vi "ARN Auswertung.vi"(8 "error in (no error)":errorcluster caption="Fehler (Eingang, kein Fehler)") -> (0 "error out":errorcluster caption="Fehler (Ausgang)")   [LabVIEW 2020, in "EPA 1065.lvlib" / "ARN Test 1065-305.lvlib"]
uses:
  ARN Test 1065-305.lvlib
  Aktion FGV ARN Daten.ctl
  Messdaten/Gewichtung (Stichprobe).ctl
  Messdaten/Messdaten.lvlib
  ARN Modus.ctl
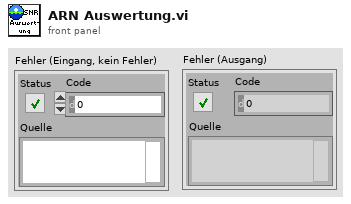
[diagram p1: front panel]
types:
  T1 = typedef "Messdaten.lvlib/Gewichtung (Stichprobe).ctl" = enum16{"Sample", "Population"}
  T2 = typedef "EPA 1065.lvlib/ARN Test 1065-305.lvlib/Aktion FGV ARN Daten.ctl" = enum16{"Lesen", "laden", "speichern", "ARN Daten", "Rohdaten", "Rohdaten löschen", "Zeitstempel", "SNR Ergebnis"}
  T3 = typedef "EPA 1065.lvlib/ARN Test 1065-305.lvlib/Allgemeine Einstellungen.ctl" = cluster{"Bearbeiter:":string, "Analysator":T4, "Komponente:":u16, "Gasflaschen Nr.:":string, "Accuracy":dbl, "Sollwert":dbl, "Modus":T5, "Pfad:":path, "Textname:":string, "CG Aufschaltzeit:":dbl, "Einheit":string, "N2 Aufschaltzeit:":dbl, "Gasflasche":T6, "Konfig Gasflasche":T7}
  T4 = typedef "System Einstellungen V2.lvlib/Analysatoren.ctl" = string
  T5 = typedef "EPA 1065.lvlib/T90 Test 1065-308.lvlib/Modus.ctl" = u16
  T6 = typedef "System Einstellungen V2.lvlib/Gasflasche Auswahl.ctl" = u16
  T7 = typedef "System Einstellungen V2.lvlib/Konfig Gasflasche.ctl" = bool
  T8 = typedef "EPA 1065.lvlib/ARN Test 1065-305.lvlib/ARN Modus.ctl" = u16
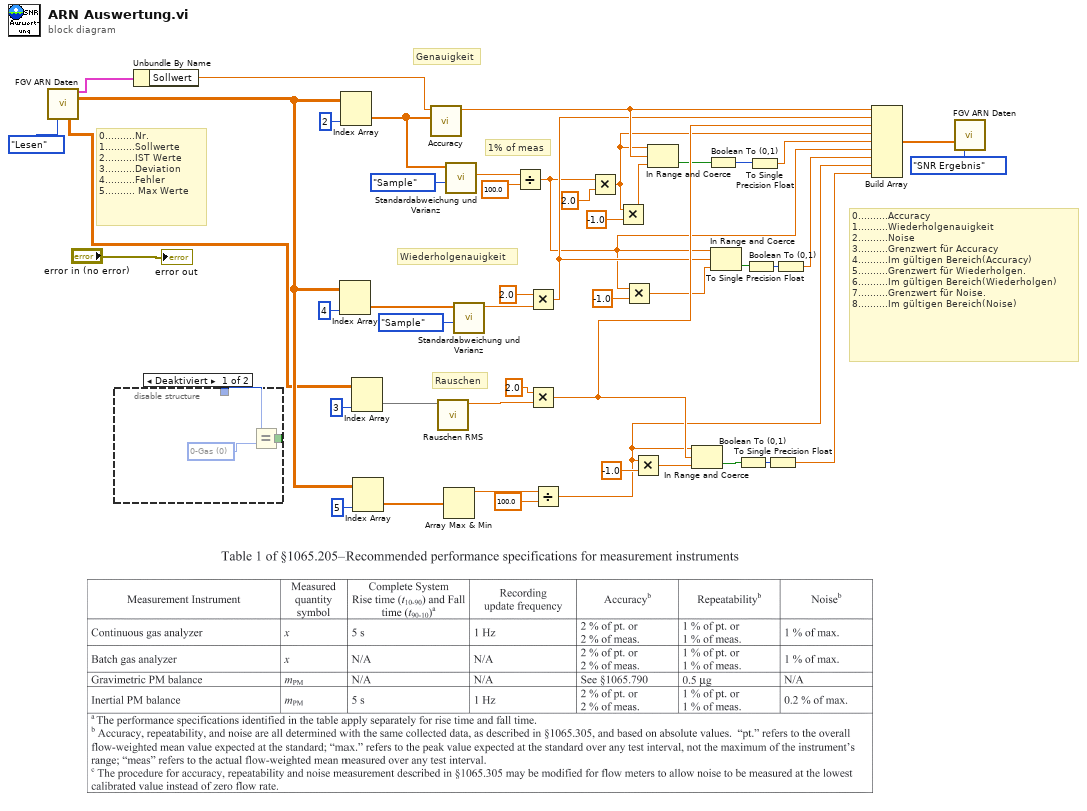
[diagram p0: block diagram]
diagram:
  # "0..........Accuracy\n1..........Wiederholgenauigkeit\n2..........Noise\n3..........Grenzwert für Accuracy\n4..........Im gültigen Bereich(Accuracy)\n5..........Grenzwert für Wiederholgen.\n6..........Im gültigen Bereich(Wiederholgen)\n7..........Grenzwert für Noise.\n8..........Im gültigen Bereich(Noise)"
  # "0..........Nr.\n1..........Sollwerte\n2..........IST Werte\n3..........Deviation\n4..........Fehler\n5.......... Max Werte"
  # "1% of meas"
  # "Rauschen"
  # "Wiederholgenauigkeit"
  # "Genauigkeit"
  n1 = call "FGV ARN Daten.vi"("Aktion"=Aktion_FGV_ARN_Daten."Lesen") -> ("ARN Konfig Daten"=w46:T3, "Rohdaten"=w35:sgl[][], "Rohdaten N2"=w2:sgl[][])  [unwired: 9 in, 3 out]
  n2 = disable-structure shown="Deaktiviert" {
    disable-tunnel: [w50 _] -> _
    disable-tunnel: _ -> [w49 _]
    frame Disabled {
      w51 = T8 0 items=["0-Gas", "CalGas", "CalGas zu PNS"] ("y")
      n3 = Equal?(x=w49, y=w51) -> (x = y?=w50:bool)
    }
    frame Enabled {
    }
  }
  n4 = Unbundle By Name(w46) -> ("Sollwert"=w45:dbl)
  n5 = Index Array(array=w35, index (col)=4 ("Deaktivierter Index (Spalte)")) -> (element=w42:sgl[])  [unwired: 1 in]
  n6 = Index Array(array=w35, index (col)=2 ("Deaktivierter Index (Spalte)")) -> (element=w27:sgl[])  [unwired: 1 in]
  n7 = Index Array(array=w2, index (col)=3 ("Deaktivierter Index (Spalte)")) -> (element=w4:sgl[])  [unwired: 1 in]
  n8 = Index Array(array=w35, index (col)=5 ("Deaktivierter Index (Spalte)")) -> (element=w34:sgl[])  [unwired: 1 in]
  n9 = call "Accuracy.vi"("Y"=w27, "Yref"=w45) -> ("Accuracy"=w21:sgl)  [unwired: 9 in]
  n10 = call "Rauschen RMS.vi"("Eingang"=w4) -> ("RMS"=w3:sgl)  [unwired: 10 in]
  n11 = Array Max & Min(array=w34) -> (max value=w33:sgl)  [unwired: 3 out]
  n12 = call "Standardabweichung und Varianz.vi"("Gewichtung (Stichprobe)"=Gewichtung_(Stichprobe)."Sample", "X"=w27) -> ("Mittelwert"=w26:sgl)  [unwired: 7 in, 2 out]
  n13 = call "Standardabweichung und Varianz.vi"("Gewichtung (Stichprobe)"=Gewichtung_(Stichprobe)."Sample", "X"=w42) -> ("Standardabweichung"=w41:sgl)  [unwired: 7 in, 2 out]
  n14 = Divide(x=w26, y=sgl 100.0) -> (x/y=w11:sgl)
  n15 = Multiply(x=sgl 2.0, y=w41) -> (x*y=w18:sgl)
  n16 = Multiply(x=sgl 2.0, y=w3) -> (x*y=w29:sgl)
  n17 = Divide(x=w33, y=sgl 100.0) -> (x/y=w9:sgl)
  n18 = Multiply(x=w11, y=sgl 2.0 ("x")) -> (x*y=w16:sgl)
  n19 = Multiply(x=w16, y=sgl -1.0) -> (x*y=w22:sgl)
  n20 = Multiply(x=w11, y=sgl -1.0) -> (x*y=w19:sgl)
  n21 = Multiply(x=w9, y=sgl -1.0) -> (x*y=w30:sgl)
  n22 = In Range and Coerce(upper limit=w16, x=w21, lower limit=w22) -> (In Range?=w15:bool)  [unwired: 1 out]
  n23 = In Range and Coerce(upper limit=w9, x=w29, lower limit=w30) -> (In Range?=w7:bool)  [unwired: 1 out]
  n24 = Boolean To (0,1)(Boolean=w15) -> (0, 1=w14:i16)
  n25 = In Range and Coerce(upper limit=w11, x=w18, lower limit=w19) -> (In Range?=w17:bool)  [unwired: 1 out]
  n26 = Boolean To (0,1)(Boolean=w7) -> (0, 1=w8:i16)
  n27 = Boolean To (0,1)(Boolean=w17) -> (0, 1=w12:i16)
  n28 = To Single Precision Float(number=w14) -> (single precision float=w13:sgl)
  n29 = To Single Precision Float(number=w8) -> (single precision float=w6:sgl)
  n30 = To Single Precision Float(number=w12) -> (single precision float=w10:sgl)
  n31 = Build Array(w21, w18, w29, w16, w13, w11, w10, w9, w6) -> (w37:sgl[])
  n32 = call "FGV ARN Daten.vi"("SNR Ergebnis"=w37, "Aktion"=Aktion_FGV_ARN_Daten."SNR Ergebnis") -> ()  [unwired: 8 in, 6 out]
  "error out" <- "error in (no error)"
